vi "LESO_open.vi"(8 "error in":errorcluster, 10 "Serial Config":T1={"Baudrate"=115200, "Word Length"=8, "Stop Bits"=0, "Parity"=0} {"Parity" items=["FT_PARITY_NONE", "FT_PARITY_ODD", "FT_PARITY_EVEN", "FT_PARITY_MARK", "FT_PARITY_SPACE"]; "Stop Bits" items=["FT_STOP_BITS_1"=0, "FT_STOP_BITS_2"=2]; "Word Length" items=["FT_BITS_7"=7, "FT_BITS_8"=8]}, 11 "LESO Name":string="LESO6") -> (0 "error out":errorcluster, 2 "Serial Number":string, 3 "Handle":u32)   [LabVIEW 2012]
doc: "Открывает соединение с устройством LESO. Настраивает параметры обмена по последовательному порту. Возвращает дескриптор соединения <B>handle</B>. Этот дескриптор должен быть использован для последующей работы с устройством.\nИспользуется драйвер <B>D2XX</B>, динамическая библиотека <B>ftd2xx.dll</B>."
uses:
  FTD2XX.dll
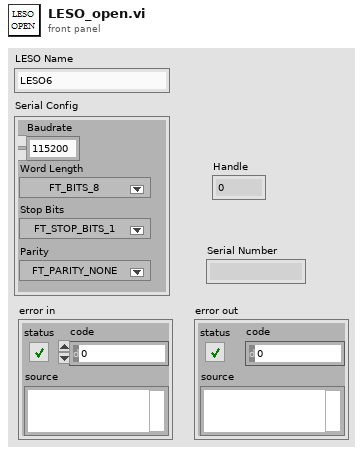
[diagram p1: front panel]
types:
  T1 = cluster{"Baudrate":u32, "Word Length":u8, "Stop Bits":u8, "Parity":u8}
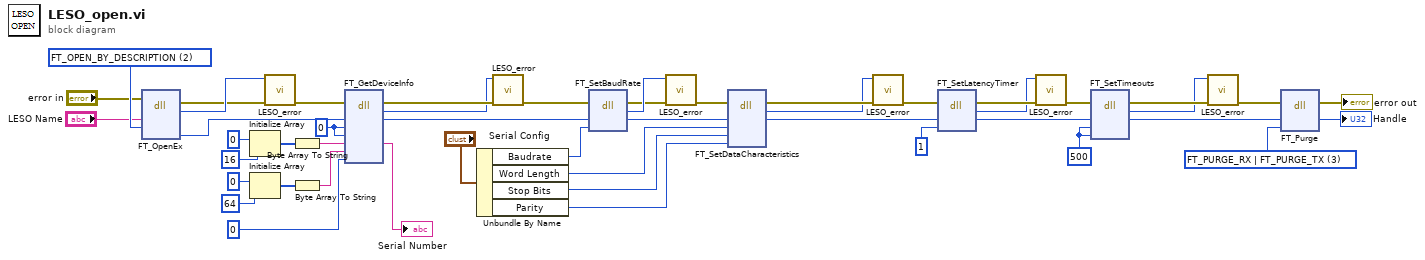
[diagram p0: block diagram]
diagram:
  w29 = u32 3 items=["FT_PURGE_RX"=1, "FT_PURGE_TX"=2, "FT_PURGE_RX | FT_PURGE_TX"=3] ("Purge Flags")
  w30 = u32 0 ("DeviceType")
  w48 = u32 2 items=["FT_OPEN_BY_SERIAL_NUMBER"=1, "FT_OPEN_BY_DESCRIPTION"=2, "FT_OPEN_BY_LOCATION"=4] ("Flags")
  w31 = u32 500 ("Read Timeout")
  n1 = dll-call lib="FTD2XX.dll" fn="FT_OpenEx"(error in="error in", "DeviceDescription"="LESO Name", "Flags"=w48) -> (error out=w3:errorcluster, "FT_Status"=w19:u32, "Handle"=w38:u32)  [unwired: 5 in, 1 out]
  n2 = Initialize Array(u8 0, 16 ("dimension size")) -> (w45:u8[])
  n3 = Initialize Array(u8 0, 64 ("dimension size")) -> (w43:u8[])
  n4 = call "LESO_error.vi"("error in"=w3, "FT_Status"=w19) -> ("error out"=w2:errorcluster)  [unwired: 9 in]
  n5 = Byte Array To String(unsigned byte array=w45) -> (string=w39:string)
  n6 = Byte Array To String(unsigned byte array=w43) -> (string=w40:string)
  n7 = dll-call lib="FTD2XX.dll" fn="FT_GetDeviceInfo"(error in=w2, "Handle"=w38, "DeviceType"=w30, "ID"=w30, "SerialNumber"=w39, "Description"=w40, "Dummy"=u32 0) -> (error out=w18:errorcluster, "FT_Status"=w16:u32, "Handle"=w36:u32, "SerialNumber"=→"Serial Number":string)  [unwired: 6 in, 1 out]
  n8 = Unbundle By Name("Serial Config") -> ("Baudrate"=w23:u32, "Word Length"=w22:u8, "Stop Bits"=w21:u8, "Parity"=w20:u8)
  n9 = call "LESO_error.vi"("error in"=w18, "FT_Status"=w16) -> ("error out"=w17:errorcluster)  [unwired: 9 in]
  n10 = dll-call lib="FTD2XX.dll" fn="FT_SetBaudRate"(error in=w17, "Handle"=w36, "BaudRate"=w23) -> (error out=w14:errorcluster, "FT_Status"=w15:u32, "Handle"=w35:u32)  [unwired: 3 in, 1 out]
  n11 = call "LESO_error.vi"("error in"=w14, "FT_Status"=w15) -> ("error out"=w13:errorcluster)  [unwired: 9 in]
  n12 = dll-call lib="FTD2XX.dll" fn="FT_SetDataCharacteristics" label="FT_SetDataCharactceristics"(error in=w13, "Handle"=w35, "WordLength"=w22, "StopBits"=w21, "Parity"=w20) -> (error out=w12:errorcluster, "FT_Status"=w10:u32, "Handle"=w34:u32)  [unwired: 5 in, 1 out]
  n13 = call "LESO_error.vi"("error in"=w12, "FT_Status"=w10) -> ("error out"=w11:errorcluster)  [unwired: 9 in]
  n14 = dll-call lib="FTD2XX.dll" fn="FT_SetLatencyTimer"(error in=w11, "Handle"=w34, "Timer"=u8 1 ("Latency Timer Value")) -> (error out=w9:errorcluster, "FT_Status"=w7:u32, "Handle"=w32:u32)  [unwired: 3 in, 1 out]
  n15 = call "LESO_error.vi"("error in"=w9, "FT_Status"=w7) -> ("error out"=w8:errorcluster)  [unwired: 9 in]
  n16 = dll-call lib="FTD2XX.dll" fn="FT_SetTimeouts"(error in=w8, "Handle"=w32, "ReadTimeout"=w31, "WriteTimeout"=w31) -> (error out=w6:errorcluster, "FT_Status"=w4:u32, "Handle"=w28:u32)  [unwired: 4 in, 1 out]
  n17 = call "LESO_error.vi"("error in"=w6, "FT_Status"=w4) -> ("error out"=w5:errorcluster)  [unwired: 9 in]
  n18 = dll-call lib="FTD2XX.dll" fn="FT_Purge"(error in=w5, "Handle"=w28, "Flags"=w29) -> (error out=→"error out":errorcluster, "Handle"=→"Handle":u32)  [unwired: 4 in, 1 out]
